vi "Test S7.vi"() -> ()   [LabVIEW 2020]
panel:
  out "Data":sgl
  out "Time":u32 format="%.0f ms"
  out "OK?":bool
  out "Read Data":u8[](array[numeric])
  in  "Datat Type":enum16{"I", "Q", "M", "D", "Count", "Timer"}(ring)
  in  "Write Byte":u8[](array[numeric])
  in  "Start Address":u16
  in  "DB block":u16
  in  "Slot":u8
  in  "Rack":u8
  in  "remote address":string="192.168.0.3"
  in  "PLC type":T1(ring)
  in  "Write":bool
  in  "Data Type":enum16{"I", "Q", "M", "D", "Count", "Timer"}(ring)=enum."Q"
  in  "count":i32=1
  in  "Start Address":u16
  in  "DB block":u16
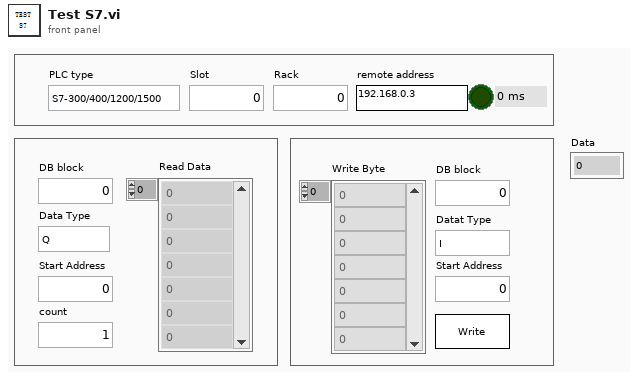
[diagram p1: front panel]
types:
  T1 = enum16{"S7-300/400/1200/1500", "S7-200", "S7-200Smart"}
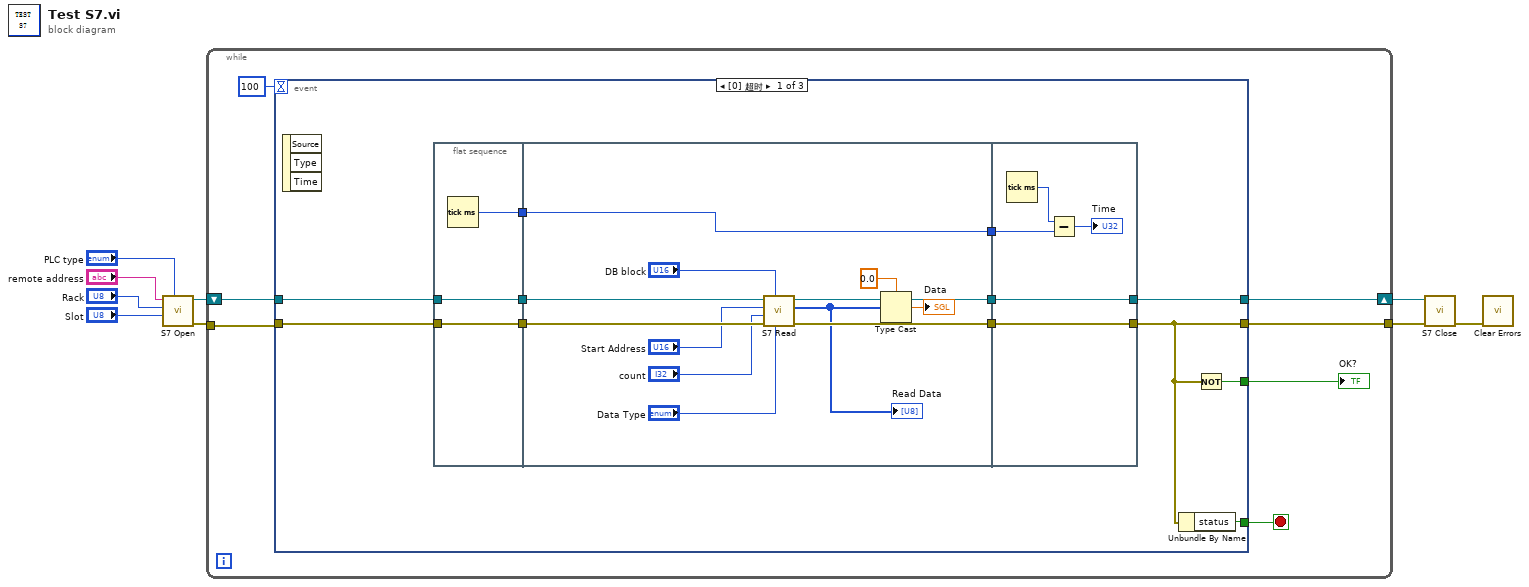
[diagram p0: block diagram]
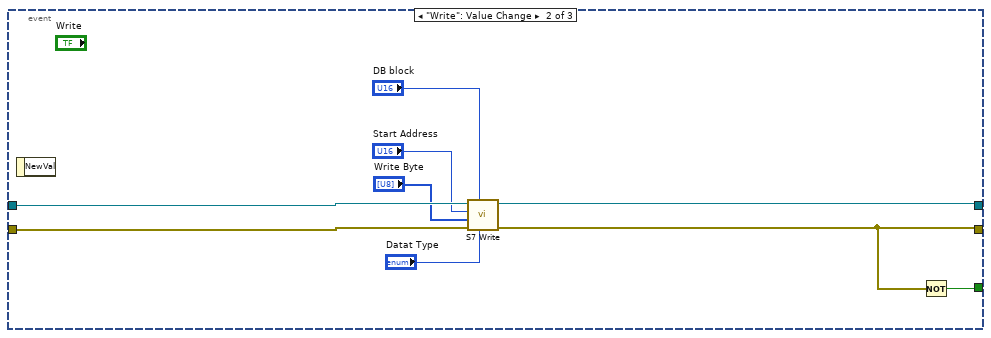
[diagram p2: hidden frame]
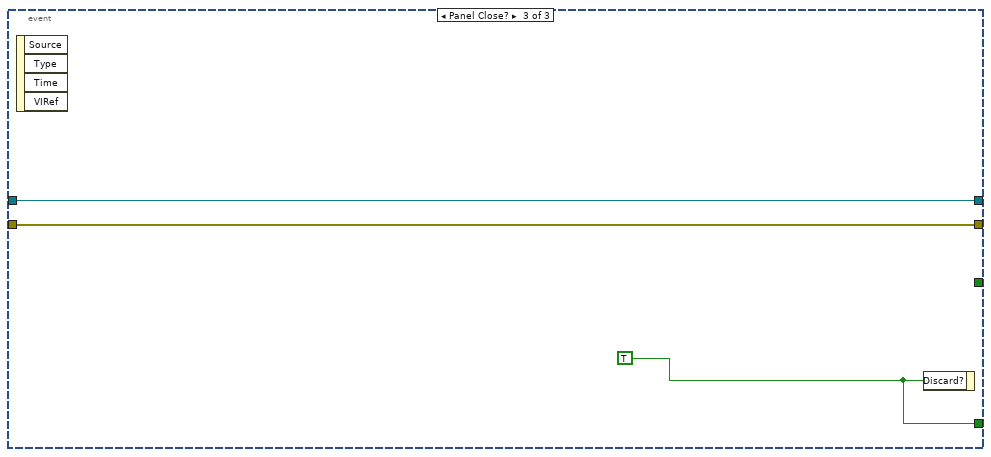
[diagram p3: hidden frame]
diagram:
  n1 = call "S7 Open.vi"("PLC type"="PLC type", "Slot"="Slot", "Rack"="Rack", "remote address"="remote address") -> ("error out"=w7:errorcluster, "TCP Out"=w9:refnum<k5>)  [unwired: 5 in, 1 out]
  n2 = while {
    shift-right: [w13] -> w8
    shift-left: w9 -> [w14]
    tunnel: w7 -> [w12]
    tunnel: [w11] -> w6
    stop <- w16 stop-if-true
    n3 = event shown="[0] 超时" {
      selector: _ -> [_ _ _]
      dyn-events: _ -> [_ _ _]
      timeout: 100 -> [_ _ _]
      tunnel: [w23 _ w60] -> w16
      tunnel: w14 -> [w28 w57 w59]
      tunnel: [w27 w56 w59] -> w13
      tunnel: w12 -> [w26 w55 w58]
      tunnel: [w24 w50 w58] -> w11
      tunnel: [w25 w49 _] -> w10
      event Timeout {
        n4 = event-data() -> ()  [unwired: 1 in, 3 out]
        n5 = flat-sequence {
          tunnel: w26 -> [w30]
          tunnel: w28 -> [w31]
          tunnel: [w31] -> w20
          tunnel: [w30] -> w19
          tunnel: [w29] -> w17
          tunnel: [w42] -> w22
          tunnel: [w36] -> w21
          tunnel: w20 -> [w43]
          tunnel: w19 -> [w41]
          tunnel: [w35] -> w18
          tunnel: w17 -> [w35]
          tunnel: [w47] -> w24
          tunnel: [w48] -> w27
          tunnel: w22 -> [w48]
          tunnel: w21 -> [w47]
          tunnel: w18 -> [w45]
          frame #0 {
            n6 = Tick Count (ms)() -> (millisecond timer value=w29:u32)
          }
          frame #1 {
            n7 = call "S7 Read.vi"("Data Type"="Data Type", "DB.NO."="DB block", "Error In"=w41, "count"="count", "StartByteAddr"="Start Address", "TCP In"=w43) -> ("error out"=w36:errorcluster, "Read Data"=w34:u8[], "TCP Out"=w42:refnum<k5>)  [unwired: 2 in, 1 out]
            "Read Data" <- w34
            n8 = Type Cast(type=sgl 0.0, x=w34) -> (*(type *) &x=→"Data":sgl)
          }
          frame #2 {
            n9 = Tick Count (ms)() -> (millisecond timer value=w46:u32)
            n10 = Subtract(x=w46, y=w45) -> (x-y=→"Time":u32)
          }
        }
        n11 = Unbundle By Name(w24) -> ("status"=w23:bool)
        n12 = Not(x=w24) -> (.not. x?=w25:bool)
      }
      event "Write": Value Change {
        n13 = event-data() -> ()  [unwired: 1 in, 1 out]
        n14 = call "S7 Write.vi"("Data Type"="Datat Type", "DB block"="DB block", "Error In"=w55, "Write Byte"="Write Byte", "Start Address"="Start Address", "TCP In"=w57) -> ("Error out"=w50:errorcluster, "TCP Out"=w56:refnum<k5>)  [unwired: 4 in]
        n15 = Not(x=w50) -> (.not. x?=w49:bool)
      }
      event Panel Close? {
        w60 = TRUE ("放弃？")
        n16 = event-data() -> ()  [unwired: 1 in, 4 out]
        n17 = event-data("Discard?"=w60) -> ()  [unwired: 1 in, 1 out]
      }
    }
    "OK?" <- w10
  }
  n18 = call "S7 Close.vi"("Error In"=w6, "TCP In"=w8) -> ("error out"=w1:errorcluster)  [unwired: 9 in]
  n19 = call <vilib>:"Clear Errors.vi"("error in (no error)"=w1) -> ()  [unwired: 5 in, 2 out]
